vi "Update Plugin Tab UI.vi"(8 "error in (no error)":errorcluster, 10 "Plugin Name":string="My Cool Plugin", 11 "CIF_UI in":refnum<class "CIF_UI.lvclass">) -> (0 "error out":errorcluster)   [LabVIEW 2021, in "CIF_UI.lvclass"]
uses:
  CIF_UI.lvclass
  CIF_UI.lvclass/CIF_UI.ctl
  Typedef/CIF_Manager_UI_Tab.ctl
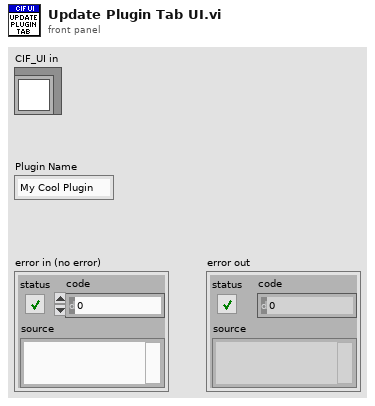
[diagram p1: front panel]
types:
  T1 = typedef "CIF_UI.lvclass/CIF_Manager_UI_Tab.ctl" = enum32{"System Management", "Channels", "Monitoring and Errors", "Plugin UI"}
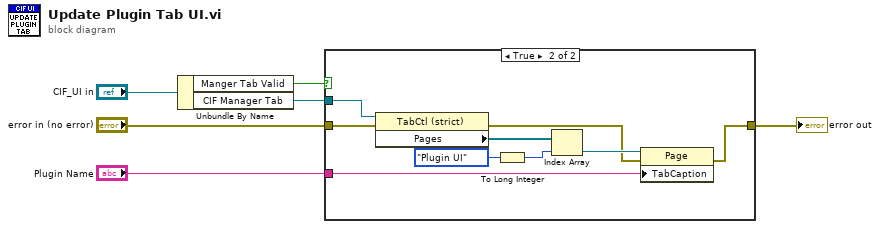
[diagram p0: block diagram]
diagram:
  n1 = Unbundle By Name("CIF_UI in") -> ("Manger Tab Valid"=w1:bool, "CIF Manager Tab"=w4:refnum<vi>)
  n2 = case shown="True" w1 {
    tunnel: "Plugin Name" -> [_ w14]
    tunnel: w4 -> [_ w13]
    tunnel: "error in (no error)" -> [w7 w10]
    tunnel: [w7 w8] -> w2
    frame False {
    }
    frame True {
      n3 = property on="Property Node" class="TabCtl (strict)"(reference=w13, error in=w10) -> (error out=w9:errorcluster, "Pages"=w16:refnum<vi>[])  [unwired: 1 out]
      n4 = To Long Integer(number=CIF_Manager_UI_Tab."Plugin UI" ("Value")) -> (32bit integer=w11:i32)
      n5 = Index Array(array=w16, index=w11) -> (element=w15:refnum<vi>)
      n6 = property class="Page"(reference=w15, error in=w9, "TabCaption"=w14) -> (error out=w8:errorcluster)  [unwired: 1 out]
    }
  }
  "error out" <- w2
